vi "quitAndRestartLabview.vi"   [LabVIEW 2017, in "ide_tools.lvlib"]
doc: "Quits and then restarts LabVIEW.\n\nIf you have unsaved files open, a dialog box prompts you to save any changes you made before the application terminates. If you cancel the dialog box, LabVIEW does not restart. \n\nThis tool is useful for restarting LabVIEW after you change the environment in a way that requires you to restart. For example, in an application that activates a license for a LabVIEW third-party add-on, you can use this method to programmatically restart LabVIEW, which then updates the status of the license."
uses:
  ide_tools.lvlib
panel:
  # "Retsrting LabVIEW. Please"
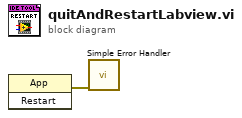
[diagram p0: block diagram]
diagram:
  n1 = invoke class="App" method="Restart"() -> (error out=w1:errorcluster)  [unwired: 3 in, 2 out]
  n2 = call <vilib>:"Simple Error Handler.vi"("error in (no error)"=w1) -> ()  [unwired: 4 in, 5 out]
